vi "GetCaseFrameNames.vi"(11 "Case reference":refnum<vi>) -> (3 "FrameNames":string[](array[string]))   [LabVIEW 2015]
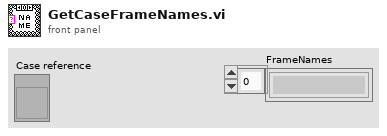
[diagram p1: front panel]
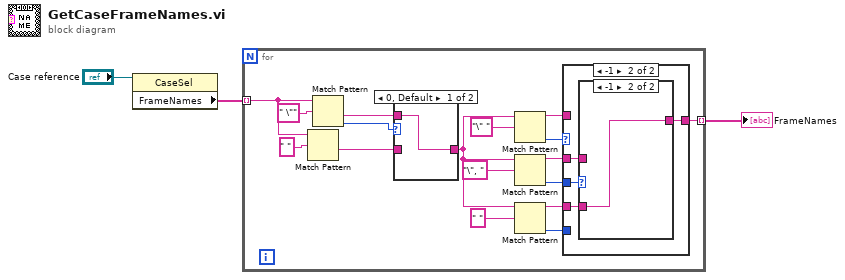
[diagram p0: block diagram]
diagram:
  n1 = property class="CaseSel"(reference="Case reference") -> ("FrameNames"=w2:string[])  [unwired: 1 in, 2 out]
  n2 = for {
    tunnel: w2 -> [w13] mode=indexing
    tunnel: [w16] -> w3 mode=indexing
    n3 = Match Pattern(string=w13, regular expression=" ") -> (after substring=w11:string)  [unwired: 1 in, 3 out]
    n4 = Match Pattern(string=w13, regular expression=" \"") -> (after substring=w14:string, offset past match=w18:i32)  [unwired: 1 in, 2 out]
    n5 = case shown="0, Default" w18 {
      tunnel: w11 -> [_ w29]
      tunnel: [w28 w29] -> w5
      tunnel: w14 -> [w28 _]
      frame 0, Default {
      }
      frame -1 {
      }
    }
    n6 = Match Pattern(string=w5, regular expression="\" ") -> (before substring=w15:string, offset past match=w17:i32)  [unwired: 1 in, 2 out]
    n7 = Match Pattern(string=w5, regular expression="\", ") -> (before substring=w9:string, offset past match=w8:i32)  [unwired: 1 in, 2 out]
    n8 = Match Pattern(string=w5, regular expression=" ") -> (before substring=w6:string, offset past match=w4:i32)  [unwired: 1 in, 2 out]
    n9 = case shown="-1" w17 {
      tunnel: w9 -> [_ w23]
      tunnel: [w21 w25] -> w16
      tunnel: w15 -> [w21 _]
      tunnel: w8 -> [_ w22]
      tunnel: w4 -> [_ _]
      tunnel: w6 -> [_ w24]
      frame 0, Default {
      }
      frame -1 {
        n10 = case shown="-1" w22 {
          tunnel: [w26 w27] -> w25
          tunnel: w24 -> [_ w27]
          tunnel: w23 -> [w26 _]
          frame 0, Default {
          }
          frame -1 {
          }
        }
      }
    }
  }
  "FrameNames" <- w3
